vi "Handle Server Request.vi"(8 "error in (no error)":errorcluster, 9 "Data":string, 10 "Method":string, 11 "Service in":refnum<class "Service.lvclass">) -> (0 "error out":errorcluster, 2 "Response":string, 3 "Service out":refnum<class "Service.lvclass">)   [LabVIEW 2024, in "Ramses Framework.lvlib" / "Service.lvclass"]
uses:
  Service.lvclass
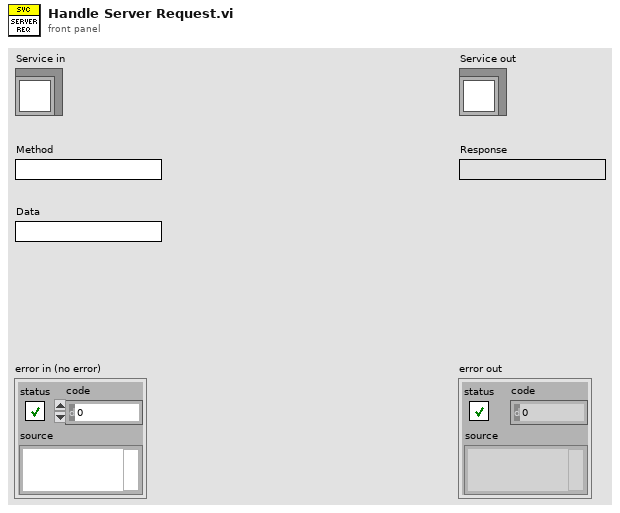
[diagram p1: front panel]
types:
  T1 = cluster{"Properties":cluster{"Name":string, "Value":string}[]}
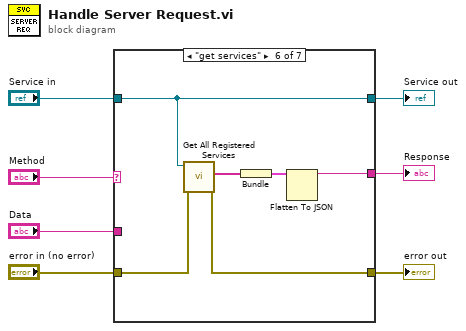
[diagram p0: block diagram]
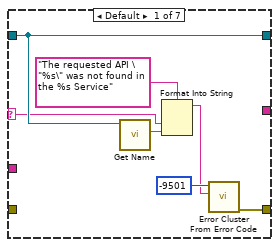
[diagram p2: hidden frame]
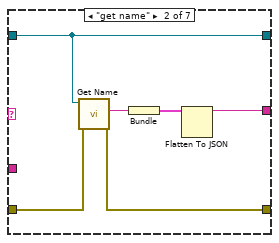
[diagram p3: hidden frame]
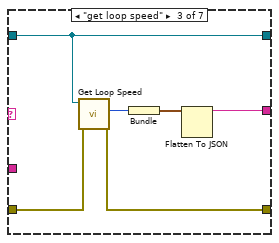
[diagram p4: hidden frame]
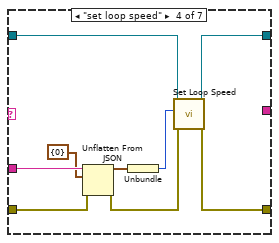
[diagram p5: hidden frame]
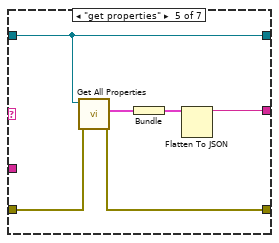
[diagram p6: hidden frame]
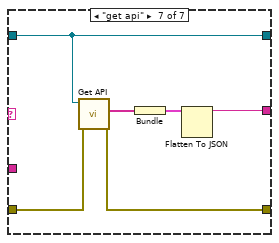
[diagram p7: hidden frame]
diagram:
  n1 = case shown="\"get services\"" "Method" {
    selector: "Method" -> [w11 _ _ _ _ _ _]
    tunnel: "Service in" -> [w12 w20 w24 w35 w40 w46 w52]
    tunnel: [w12 w20 w24 w34 w40 w46 w52] -> w6
    tunnel: "error in (no error)" -> [_ w16 w23 w29 w39 w44 w50]
    tunnel: [w14 w15 w22 w33 w38 w43 w49] -> w4
    tunnel: [_ w17 w25 _ w41 w47 w53] -> w2
    tunnel: "Data" -> [_ _ _ w32 _ _ _]
    frame Default {
      n2 = call "Get Name.vi"("Service in"=w12) -> ("Name"=w9:string)  [unwired: 8 in, 2 out]
      n3 = Format Into String(format string="The requested API \"%s\" was not found in the %s Service" ("error message (\"\")"), w11, w9) -> (resulting string=w8:string)  [unwired: 2 in, 1 out]
      n4 = call <vilib>:"Error Cluster From Error Code.vi"("error message (\"\")"=w8, "error code (0)"=-9501) -> ("error out"=w14:errorcluster)  [unwired: 7 in]
    }
    frame "get name" {
      n5 = call "Get Name.vi"("error in (no error)"=w16, "Service in"=w20) -> ("error out"=w15:errorcluster, "Name"=w19:string)  [unwired: 7 in, 1 out]
      n6 = Bundle("Name"=w19) -> (w18:cluster{"Name":string})  [unwired: 1 in]
      n7 = Flatten To JSON(anything=w18) -> (JSON string=w17:string)  [unwired: 2 in, 1 out]
    }
    frame "get loop speed" {
      n8 = call "Get Loop Speed.vi"("error in (no error)"=w23, "Service in"=w24) -> ("error out"=w22:errorcluster, "Loop Speed"=w21:i32)  [unwired: 7 in, 1 out]
      n9 = Bundle("Loop Speed"=w21) -> (w26:cluster{"Loop Speed":i32})  [unwired: 1 in]
      n10 = Flatten To JSON(anything=w26) -> (JSON string=w25:string)  [unwired: 2 in, 1 out]
    }
    frame "set loop speed" {
      n11 = Unflatten From JSON(JSON string=w32, type and defaults=cluster{"Loop Speed":i32} {"Loop Speed"=0}, error in (no error)=w29) -> (value=w28:cluster{"Loop Speed":i32}, error out=w30:errorcluster)  [unwired: 4 in]
      n12 = Unbundle(w28) -> ("Loop Speed"=w27:i32)
      n13 = call "Set Loop Speed.vi"("error in (no error)"=w30, "Loop Speed"=w27, "Service in"=w35) -> ("error out"=w33:errorcluster, "Service out"=w34:refnum<class "Service.lvclass">)  [unwired: 7 in]
    }
    frame "get properties" {
      n14 = call "Get All Properties.vi"("error in (no error)"=w39, "Service in"=w40) -> ("error out"=w38:errorcluster, "Properties"=w36:cluster{"Name":string, "Value":string}[])  [unwired: 7 in, 1 out]
      n15 = Bundle("Properties"=w36) -> (w37:T1)  [unwired: 1 in]
      n16 = Flatten To JSON(anything=w37) -> (JSON string=w41:string)  [unwired: 2 in, 1 out]
    }
    frame "get services" {
      n17 = call "Get All Registered Services.vi"("error in (no error)"=w44, "Service in"=w46) -> ("error out"=w43:errorcluster, "Services"=w45:string[])  [unwired: 7 in, 1 out]
      n18 = Bundle("Services"=w45) -> (w42:cluster{"Services":string[]})  [unwired: 1 in]
      n19 = Flatten To JSON(anything=w42) -> (JSON string=w47:string)  [unwired: 2 in, 1 out]
    }
    frame "get api" {
      n20 = call-dynamic "Get API.vi"("error in (no error)"=w50, "Service in"=w52) -> ("error out"=w49:errorcluster, "API"=w51:string[])  [unwired: 7 in, 1 out]
      n21 = Bundle("API"=w51) -> (w48:cluster{"API":string[]})  [unwired: 1 in]
      n22 = Flatten To JSON(anything=w48) -> (JSON string=w53:string)  [unwired: 2 in, 1 out]
    }
  }
  "error out" <- w4
  "Service out" <- w6
  "Response" <- w2
